vi "FoodPlane.vi"() -> ()   [LabVIEW 2013]
uses:
  InfoTable.lvclass
  FoodBase.lvclass
panel:
  out "布尔":bool
  in  "价格(小于等于）":dbl
  in  "OK":bool
  in  "名称":string
  out "?":i32(listbox)
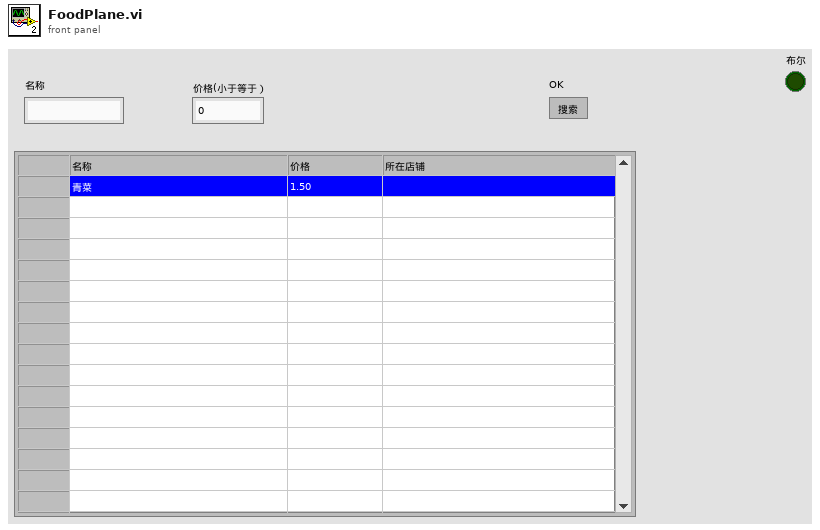
[diagram p1: front panel]
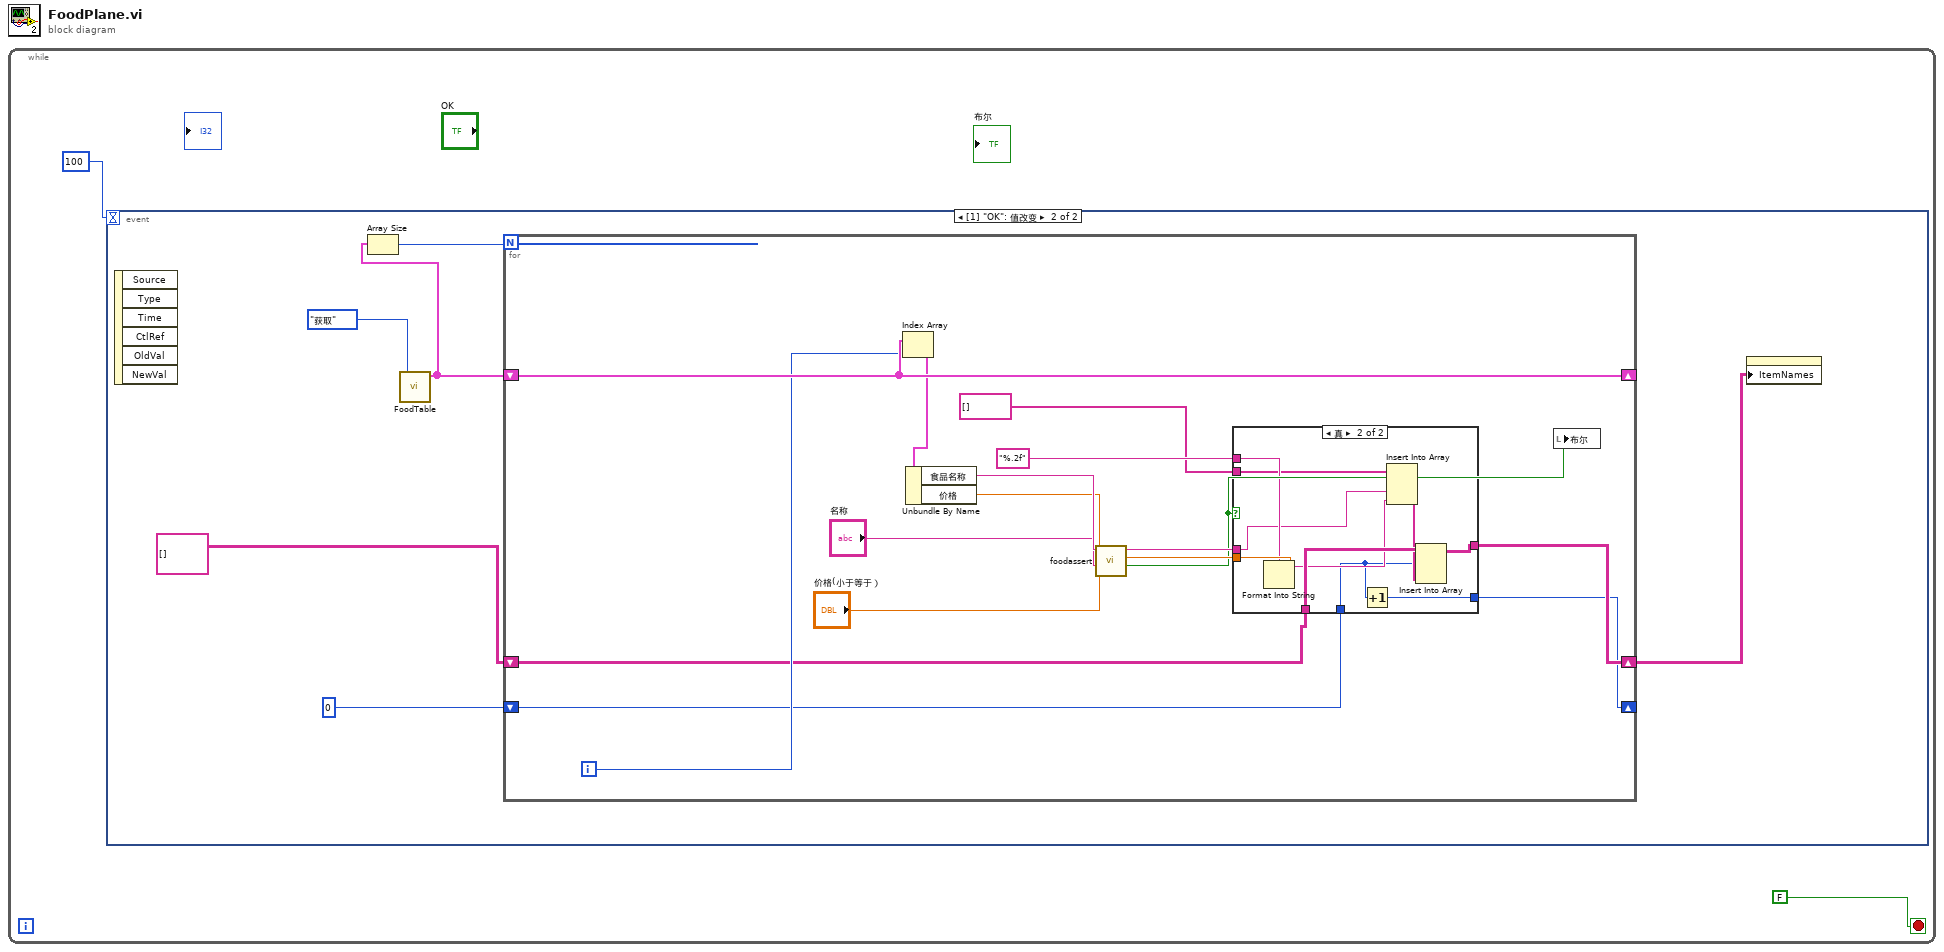
[diagram p0: block diagram]
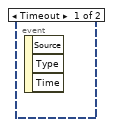
[diagram p2: hidden frame]
diagram:
  n1 = while {
    stop <- FALSE stop-if-true
    n2 = event shown="[1] \"OK\": 值改变" {
      selector: _ -> [_ _]
      dyn-events: _ -> [_ _]
      timeout: 100 -> [_ _]
      event Timeout {
        n3 = event-data() -> ()  [unwired: 1 in, 3 out]
      }
      event "OK": Value Change {
        n4 = event-data() -> ()  [unwired: 1 in, 6 out]
        n5 = call "FoodTable.vi"("枚举"=enum16{"保存", "获取", "清空", "插入", "删除", "查询"}."获取") -> ("数组"=w6:cluster{"ID":dbl, "食品名称":string, "价格":dbl}[])  [unwired: 4 in, 2 out]
        n6 = Array Size(array=w6) -> (size(s)=w7:i32)
        n7 = for {
          N: w7 -> [_]
          shift-right: [w24] -> _
          shift-left: w6 -> [w24]
          shift-right: [w16] -> w4
          shift-left: string[][] [] ("数组") -> [w17]
          shift-right: [w10] -> _
          shift-left: 0 -> [w11]
          i -> [w22]
          n8 = Index Array(array=w24, index=w22) -> (element=w23:cluster{"ID":dbl, "食品名称":string, "价格":dbl})
          n9 = Unbundle By Name(w23) -> ("食品名称"=w21:string, "价格"=w20:dbl)
          n10 = call "foodassert.vi"("价格(小于等于） 2"="价格(小于等于）", "名称 2"="名称", "价格"=w20, "食品名称"=w21) -> ("正确"=w9:bool, "价格(小于等于） 3"=w15:dbl, "名称 3"=w12:string)  [unwired: 5 in]
          n11 = case shown="真" w9 {
            tunnel: w17 -> [w26 w34]
            tunnel: [w26 w29] -> w16
            tunnel: w15 -> [_ w36]
            tunnel: "%.2f" ("格式字符串") -> [_ w35]
            tunnel: string[] [] -> [_ w33]
            tunnel: w12 -> [_ w32]
            tunnel: w11 -> [w25 w28]
            tunnel: [w25 w27] -> w10
            frame False {
            }
            frame True {
              n12 = Format Into String(format string=w35, w36) -> (resulting string=w31:string)  [unwired: 2 in, 1 out]
              n13 = Increment(x=w28) -> (x+1=w27:i32)
              n14 = Insert Into Array(array=w33, new element #1=w32, new element #2=w31) -> (w30:string[])  [unwired: 1 in]
              n15 = Insert Into Array(array=w34, index (row)=w28, new element=w30) -> (w29:string[][])  [unwired: 1 in]
            }
          }
          n16 = local write "布尔"(w9) -> ()
        }
        n17 = property class="MCListbox (严格)"("ItemNames"=w4) -> ()  [unwired: 2 in, 2 out]
      }
    }
  }
